vi "Do.vi"(8 "error in (no error)":errorcluster, 10 "Actor in":refnum<class "Actor.lvclass">, 11 "AEUpdate Msg":refnum<class "AEUpdate Msg.lvclass">) -> (0 "error out":errorcluster, 2 "Actor out":refnum<class "Actor.lvclass">)   [LabVIEW 2016, in "PVClient-Example.lvlib" / "AEUpdate Msg.lvclass"]
doc: "(<B>Filename</B>: Actor Framework.lvlib:Message.lvclass:Do.vi)\n\nDefines what a message does when it is received by an actor. Generally, a message instructs an actor to invoke one of its methods.\n\nBy default, this method does nothing. A child class must override it to define behavior. Create a child class by using the Actor Framework Message Maker dialog box."
uses:
  AEUpdate Msg.lvclass
  C:/User/Brand/LVP/CSPP-Dev/Packages/CSPP_Core/Actors/CS++PVMonitor Messages/CS++AEUpdate Msg/CS++AEUpdate Msg.lvclass
  <vilib>/ActorFramework/Actor/Actor.lvclass
  PVClient-Example/PVClient-Example.lvclass
  C:/Program Files (x86)/National Instruments/LabVIEW 2016/vi.lib/ActorFramework/Actor/Actor.lvclass
  CSPP_Core/Actors/CS++PVMonitor Messages/CS++AEUpdate Msg/CS++AEUpdate Msg.lvclass/CS++AEUpdate Msg.ctl
  CSPP_Core/Classes/CS++ProcessVariables/AlarmEvent/AE.lvclass
  CSPP_Core/Actors/CS++PVMonitor Messages/CS++AEUpdate Msg/CS++AEUpdate Msg.lvclass
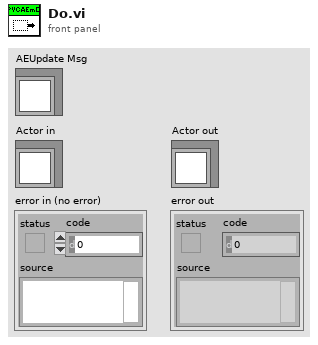
[diagram p1: front panel]
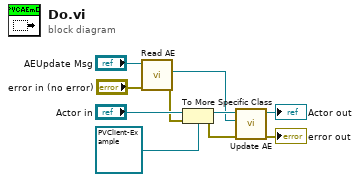
[diagram p0: block diagram]
diagram:
  n1 = call "Read AE.vi"("error in (no error)"="error in (no error)", "CS++AEUpdate Msg in"="AEUpdate Msg") -> ("error out"=w5:errorcluster, "AE"=w3:refnum<class "AE.lvclass">)  [unwired: 7 in, 1 out]
  n2 = To More Specific Class(target class=refnum<class "PVClient-Example.lvclass"> refnum ("PVClient-Example.lvlib:PVClient-Example.lvclass"), reference="Actor in", error in=w5) -> (specific class reference=w7:refnum<class "PVClient-Example.lvclass">, error out=w4:errorcluster)
  n3 = call "Update AE.vi"("error in (no error)"=w4, "AE"=w3, "PVClient-Example in"=w7) -> ("error out"=→"error out":errorcluster, "PVClient-Example out"=→"Actor out":refnum<class "PVClient-Example.lvclass">)  [unwired: 7 in]
